vi "Ft to Encoder Velocity.vi"(11 "ft/s":dbl) -> (3 "v":dbl)   [LabVIEW 2019]
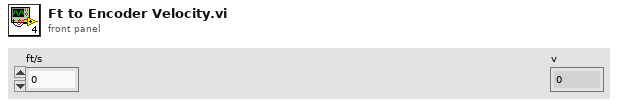
[diagram p1: front panel]
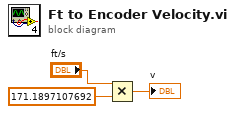
[diagram p0: block diagram]
diagram:
  n1 = Multiply(x="ft/s", y=171.1897107692) -> (x*y=→"v":dbl)
